vi "Comanament_States2.vi"(6 "Emergencia":bool, 7 "ReseUpDown":bool caption="ResetUpDown", 9 "Entradas_Botones":T1) -> (0 "Active_motor":bool, 3 "Salidas_mando":T2={"HI_down"=TRUE, " LO_down"=TRUE, "HI_up"=TRUE, "*"=TRUE, " LO_up"=TRUE, " start"=TRUE, " Ensayo_down"=TRUE, " Ensayo_up"=TRUE})   [LabVIEW 2017]
panel:
  out "number":u32
  in  "Variables_mando":T2={"HI_down"=TRUE, " LO_down"=TRUE, "HI_up"=TRUE, "*"=TRUE, " LO_up"=TRUE, " start"=TRUE, " Ensayo_down"=TRUE, " Ensayo_up"=TRUE}
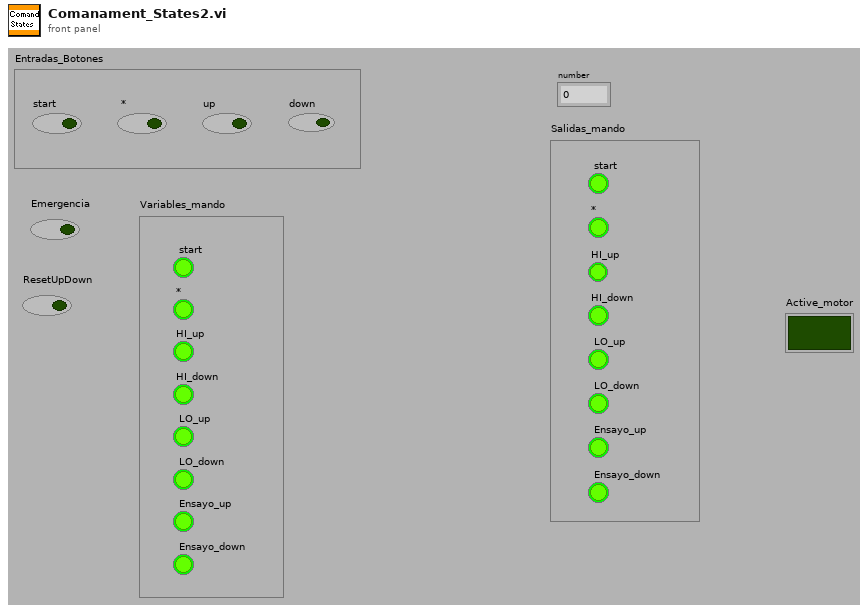
[diagram p1: front panel]
types:
  T1 = cluster{"start":bool, " *":bool, "up":bool, "down":bool}
  T2 = cluster{"HI_down":bool, " LO_down":bool, "HI_up":bool, "*":bool, " LO_up":bool, " start":bool, " Ensayo_down":bool, " Ensayo_up":bool}
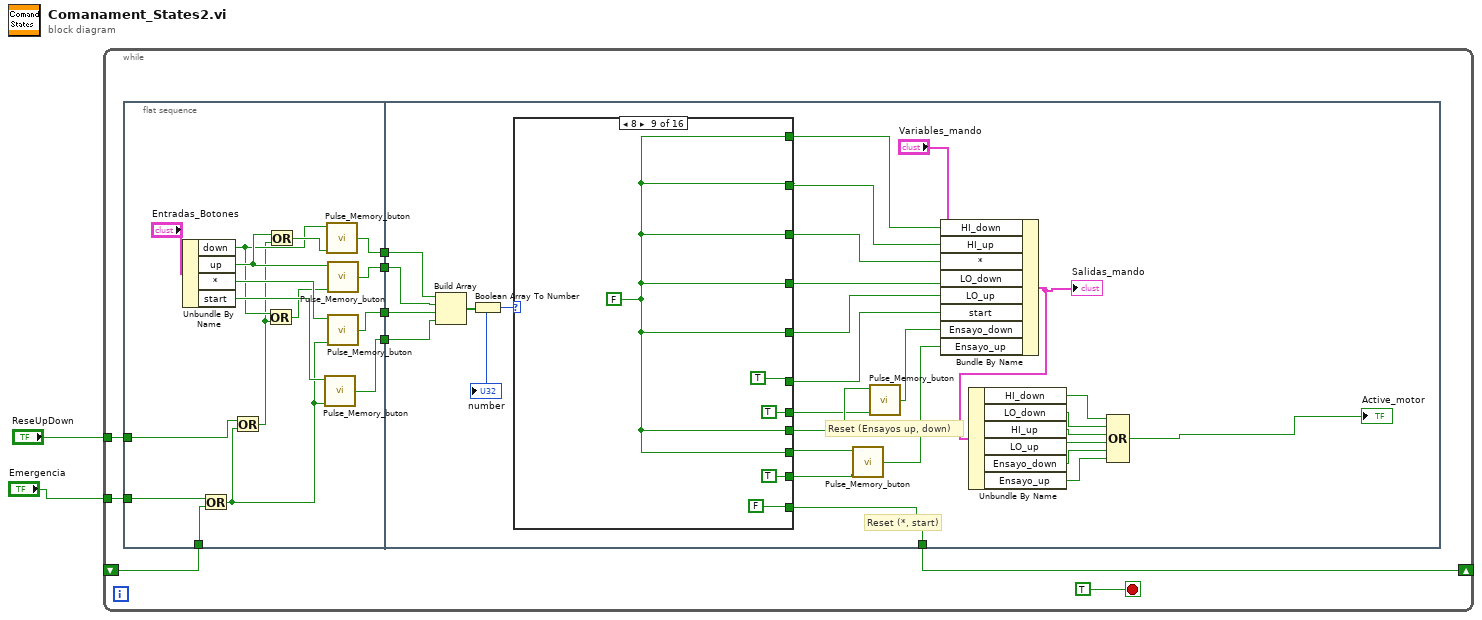
[diagram p0: block diagram]
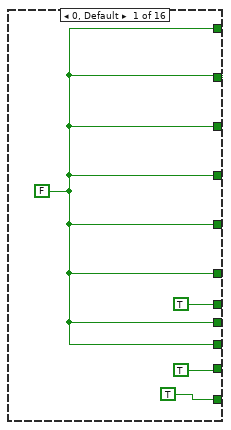
[diagram p2: hidden frame]
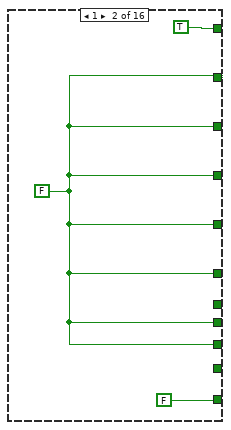
[diagram p3: hidden frame]
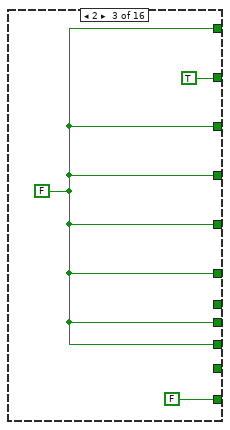
[diagram p4: hidden frame]
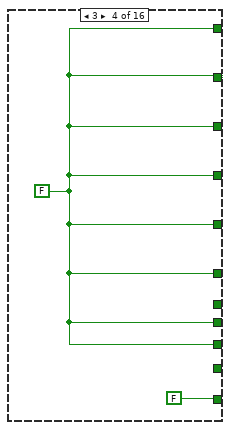
[diagram p5: hidden frame]
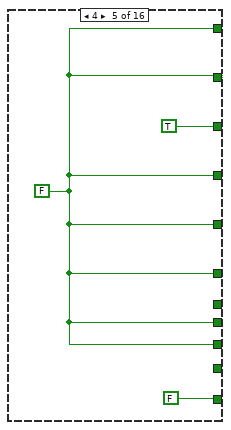
[diagram p6: hidden frame]
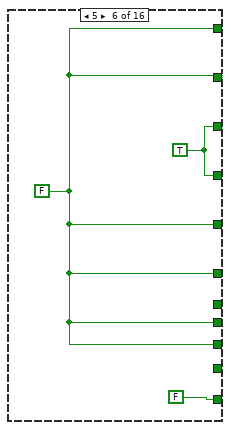
[diagram p7: hidden frame]
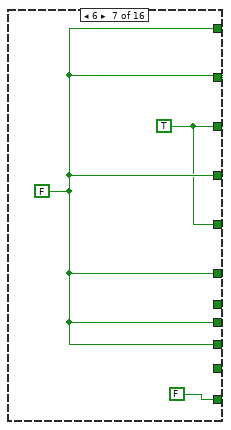
[diagram p8: hidden frame]
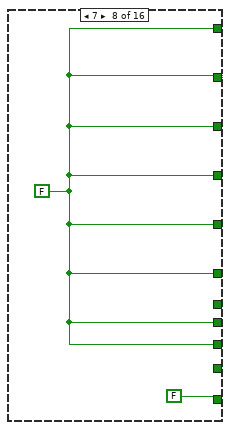
[diagram p9: hidden frame]
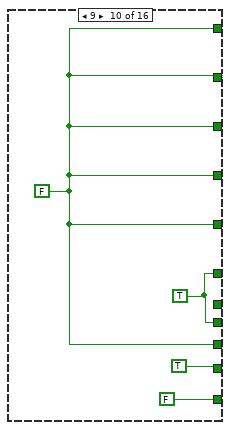
[diagram p10: hidden frame]
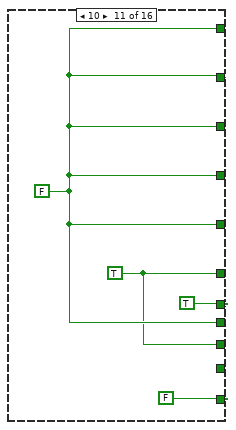
[diagram p11: hidden frame]
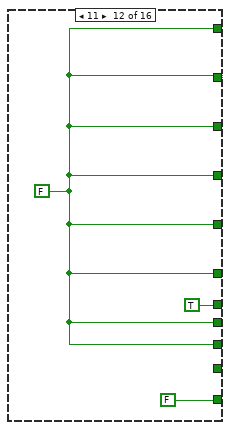
[diagram p12: hidden frame]
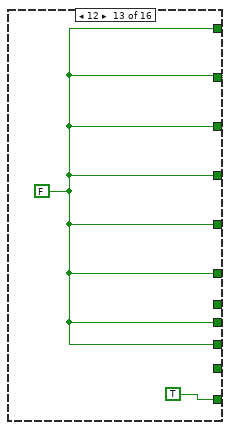
[diagram p13: hidden frame]
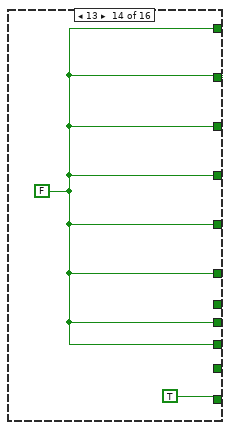
[diagram p14: hidden frame]
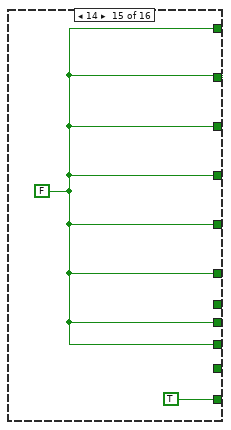
[diagram p15: hidden frame]
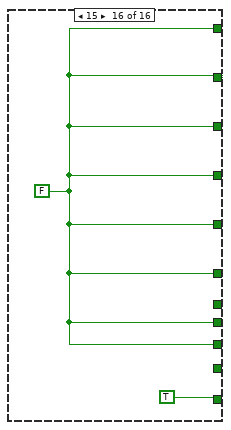
[diagram p16: hidden frame]
diagram:
  n1 = while {
    shift-right: [w5] -> _
    shift-left: _ -> [w6]
    tunnel: "Emergencia" -> [w4]
    tunnel: "ReseUpDown" -> [w3]
    stop <- TRUE stop-if-true
    n2 = flat-sequence {
      tunnel: [w27] -> w10
      tunnel: [w26] -> w9
      tunnel: w6 -> [w20]
      tunnel: [w21] -> w8
      tunnel: [w22] -> w7
      tunnel: w4 -> [w15]
      tunnel: w3 -> [w14]
      tunnel: w10 -> [w47]
      tunnel: w9 -> [w46]
      tunnel: [w45] -> w5
      tunnel: w8 -> [w41]
      tunnel: w7 -> [w40]
      frame #0 {
        n3 = Unbundle By Name("Entradas_Botones") -> ("down"=w16:bool, "up"=w17:bool, "*"=w24:bool, "start"=w23:bool)
        n4 = Or(x=w15, y=w20) -> (x .or. y?=w13:bool)
        n5 = Or(x=w14, y=w13) -> (x .or. y?=w12:bool)
        n6 = Or(x=w16, y=w12) -> (x .or. y?=w18:bool)
        n7 = Or(x=w17, y=w12) -> (x .or. y?=w19:bool)
        n8 = call "Pulse_Memory_buton.vi"("Reset"=w13, "Pulse"=w23) -> ("Memory"=w26:bool)  [unwired: 4 in]
        n9 = call "Pulse_Memory_buton.vi"("Reset"=w19, "Pulse"=w16) -> ("Memory"=w21:bool)  [unwired: 4 in]
        n10 = call "Pulse_Memory_buton.vi"("Reset"=w18, "Pulse"=w17) -> ("Memory"=w22:bool)  [unwired: 4 in]
        n11 = call "Pulse_Memory_buton.vi"("Reset"=w13, "Pulse"=w24) -> ("Memory"=w27:bool)  [unwired: 4 in]
      }
      frame #1 {
        # "Reset (Ensayos up, down)"
        # "Reset (*, start)"
        n12 = Build Array(w41, w40, w47, w46) -> (w44:bool[])
        n13 = Boolean Array To Number(Boolean array=w44) -> (number=w55:u32)
        "number" <- w55
        n14 = case shown="8" w55 {
          tunnel: [w59 TRUE w65 w67 w70 w73 w76 w78 w83 w87 w89 w94 w96 w98 w100 w102] -> w53
          tunnel: [w59 w61 TRUE w67 w70 w73 w76 w78 w83 w87 w89 w94 w96 w98 w100 w102] -> w52
          tunnel: [w59 w61 w65 w67 TRUE w72 w75 w78 w83 w87 w89 w94 w96 w98 w100 w102] -> w51
          tunnel: [w59 w61 w65 w67 w70 w72 w76 w78 w83 w87 w89 w94 w96 w98 w100 w102] -> w50
          tunnel: [w59 w61 w65 w67 w70 w73 w76 w78 w83 w87 w88 w94 w96 w98 w100 w102] -> w30
          tunnel: [w59 w61 w65 w67 w70 w73 w75 w78 w83 w87 w89 w94 w96 w98 w100 w102] -> w49
          tunnel: [w59 w61 w65 w67 w70 w73 w76 w78 w83 w86 w89 w94 w96 w98 w100 w102] -> w43
          tunnel: [w59 w61 w65 w67 w70 w73 w76 w78 TRUE w86 w88 w94 w96 w98 w100 w102] -> w48
          tunnel: [TRUE FALSE FALSE FALSE FALSE FALSE FALSE FALSE FALSE FALSE FALSE FALSE TRUE TRUE TRUE TRUE] -> w45
          tunnel: [TRUE _ _ _ _ _ _ _ TRUE _ TRUE TRUE _ _ _ _] -> w32
          tunnel: [TRUE _ _ _ _ _ _ _ TRUE TRUE _ _ _ _ _ _] -> w29
          frame 0, Default {
            w59 = FALSE
          }
          frame 1 {
            w61 = FALSE
          }
          frame 2 {
            w65 = FALSE
          }
          frame 3 {
            w67 = FALSE
          }
          frame 4 {
            w70 = FALSE
          }
          frame 5 {
            w72 = TRUE
            w73 = FALSE
          }
          frame 6 {
            w75 = TRUE
            w76 = FALSE
          }
          frame 7 {
            w78 = FALSE
          }
          frame 8 {
            w83 = FALSE
          }
          frame 9 {
            w86 = TRUE
            w87 = FALSE
          }
          frame 10 {
            w88 = TRUE
            w89 = FALSE
          }
          frame 11 {
            w94 = FALSE
          }
          frame 12 {
            w96 = FALSE
          }
          frame 13 {
            w98 = FALSE
          }
          frame 14 {
            w100 = FALSE
          }
          frame 15 {
            w102 = FALSE
          }
        }
        n15 = call "Pulse_Memory_buton.vi"("Reset"=w29, "Pulse"=w30) -> ("Memory"=w28:bool)  [unwired: 4 in]
        n16 = call "Pulse_Memory_buton.vi"("Reset"=w32, "Pulse"=w43) -> ("Memory"=w42:bool)  [unwired: 4 in]
        n17 = Bundle By Name(cluster="Variables_mando", "HI_down"=w53, "HI_up"=w52, "*"=w51, "LO_down"=w50, "LO_up"=w49, "start"=w48, "Ensayo_down"=w42, "Ensayo_up"=w28) -> (w39:T2)
        "Salidas_mando" <- w39
        n18 = Unbundle By Name(w39) -> ("HI_down"=w38:bool, "LO_down"=w37:bool, "HI_up"=w36:bool, "LO_up"=w35:bool, "Ensayo_down"=w34:bool, "Ensayo_up"=w33:bool)
        n19 = Compound Arithmetic op=OR(w38, w37, w36, w35, w34, w33) -> (→"Active_motor":bool)
      }
    }
  }
